vi "AE_Continuous_All.vi"() -> ()   [LabVIEW 2012]
uses:
  <vilib>/DAQmx/read.llb/DAQmx Read (Analog 1D Wfm NChan NSamp).vi
  <vilib>/DAQmx/create/channels.llb/DAQmx Create Channel (AI-Voltage-Basic).vi
  <vilib>/DAQmx/configure/timing.llb/DAQmx Timing (Sample Clock).vi
  <vilib>/DAQmx/miscellaneous.llb/DAQmx Fill In Error Info.vi
panel:
  in  "Physical Channel":tag="Dev1/ai7"
  in  "Gain":u16(ring)=1 items=["20 dB", "40 dB", "60 dB"]
  in  "stop":bool
  in  "Test Name":string="test"
  in  "Storage Directory":path=path "C:/Users/User/Desktop/Users_2013-2014/Michael Rossol"
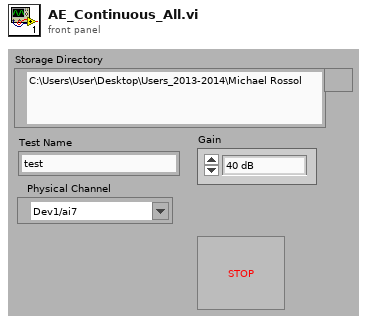
[diagram p1: front panel]
types:
  T1 = enum16{"open", "open or create", "create or replace", "create", "open (read only)"}
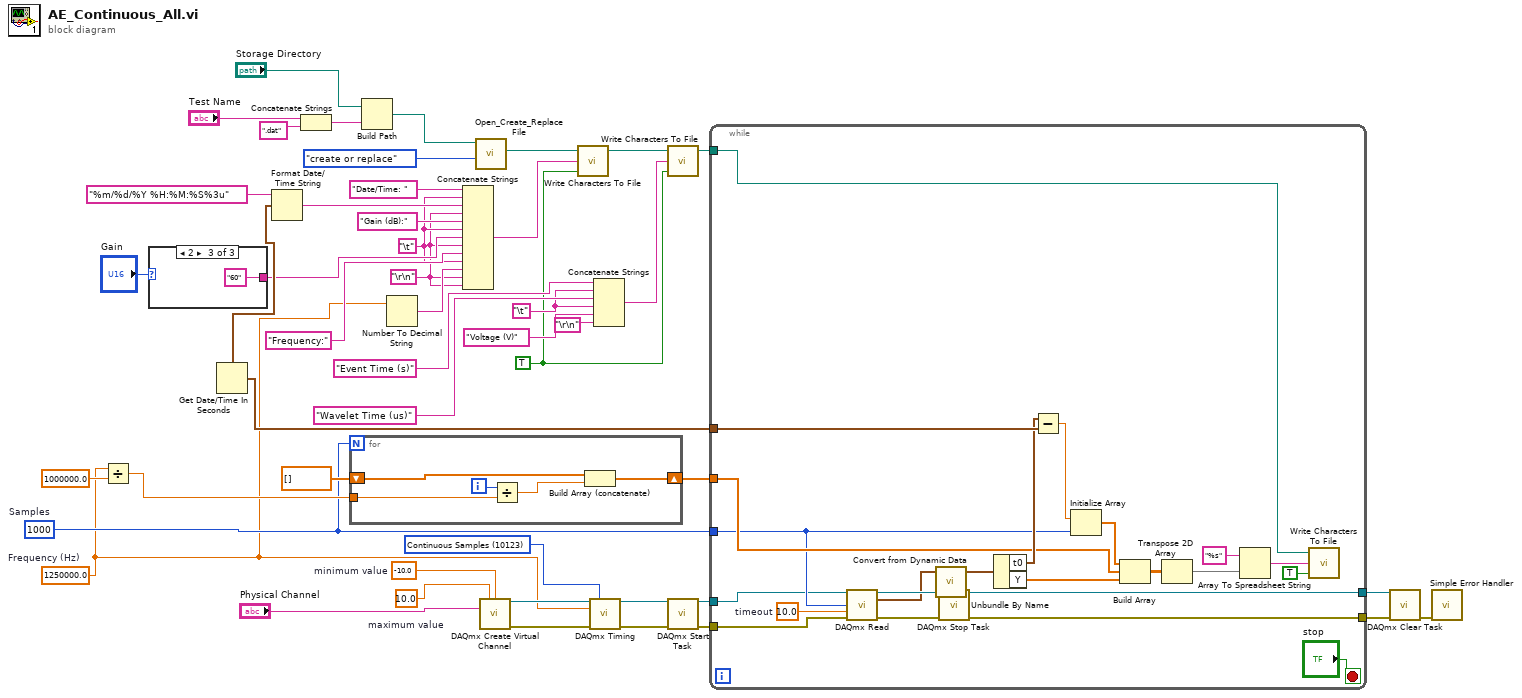
[diagram p0: block diagram]
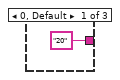
[diagram p2: hidden frame]
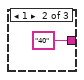
[diagram p3: hidden frame]
diagram:
  w2 = 1000  # Samples
  w20 = -10.0  # minimum value
  w21 = 10.0  # maximum value
  w17 = 10123 items=["Finite Samples"=10178, "Continuous Samples"=10123] ("sample mode")
  w31 = "\t"
  w1 = 1250000.0  # Frequency (Hz)
  w9 = "\t"
  w7 = "\r\n"
  w28 = TRUE ("append to file? (new file:F)")
  n1 = Divide(x=w1, y=1000000.0) -> (x/y=w34:dbl)
  n2 = case shown="2" "Gain" {
    tunnel: ["20" ("string") "40" ("string") "60" ("string")] -> w22
    frame 0, Default {
    }
    frame 1 {
    }
    frame 2 {
    }
  }
  n3 = Get Date/Time In Seconds() -> (seconds since 1Jan1904=w35:timestamp)
  n4 = Format Date/Time String(time format string (%c)="%m/%d/%Y %H:%M:%S%3u", seconds (now)=w35) -> (date/time string=w37:string)  [unwired: 1 in]
  n5 = Concatenate Strings("Test Name", ".dat" ("string")) -> (w40:string)
  n6 = for {
    N: w2 -> [_]
    shift-right: [w54] -> w13
    shift-left: dbl[] [] -> [w55]
    tunnel: w34 -> [w51]
    i -> [w53]
    n7 = Divide(x=w53, y=w51) -> (x/y=w52:dbl)
    n8 = Build Array (concatenate)(w55, w52) -> (w54:dbl[])
  }
  n9 = Build Path(base path="Storage Directory", name or relative path=w40) -> (appended path=w38:path)
  n10 = Number To Decimal String(number=w1) -> (decimal integer string=w8:string)  [unwired: 1 in]
  n11 = Concatenate Strings("Date/Time: ", w9, w37, w7, "Gain (dB):" ("string"), w9, w22, w7, "Frequency:" ("string"), w9, w8, w7, w7) -> (w47:string)
  n12 = call <vilib>:"Open_Create_Replace File.vi"("function (open:0)"=T1."create or replace", "file path"=w38) -> ("new file path"=w43:path)  [unwired: 6 in, 3 out]
  n13 = call-poly <vilib>:"DAQmx Create Virtual Channel.vi"("maximum value"=w21, "minimum value"=w20, "physical channels"="Physical Channel") -> ("task out"=w19:refnum<k21>, "error out"=w18:errorcluster)  [unwired: 11 in]
  n14 = call <vilib>:"Write Characters To File.vi"("append to file? (new file:F)"=w28, "character string"=w47, "file path (dialog if empty)"=w43) -> ("new file path (Not A Path if cancelled)"=w26:path)  [unwired: 2 in]
  n15 = call-poly <vilib>:"DAQmx Timing.vi"("task/channels in"=w19, "sample mode"=w17, "rate"=w1, "error in"=w18) -> ("task out"=w5:refnum<k21>, "error out"=w6:errorcluster)  [unwired: 10 in]
  n16 = Concatenate Strings("Event Time (s)" ("string"), w31, "Wavelet Time (us)" ("string"), w31, "Voltage (V)" ("string"), "\r\n") -> (w27:string)
  n17 = call <vilib>:"Write Characters To File.vi"("append to file? (new file:F)"=w28, "character string"=w27, "file path (dialog if empty)"=w26) -> ("new file path (Not A Path if cancelled)"=w25:path)  [unwired: 2 in]
  n18 = call <vilib>:"DAQmx Start Task.vi"("task/channels in"=w5, "error in"=w6) -> ("task out"=w4:refnum<k21>, "error out"=w3:errorcluster)  [unwired: 12 in]
  n19 = while {
    tunnel: w25 -> [w75]
    tunnel: w2 -> [w59]
    tunnel: w35 -> [w72]
    tunnel: w13 -> [w66]
    tunnel: [w62] -> w15
    tunnel: [w61] -> w14
    tunnel: w4 -> [w57]
    tunnel: w3 -> [w56]
    stop <- "stop" stop-if-true
    w65 = 10.0  # timeout
    n20 = call-poly <vilib>:"DAQmx Read.vi"("task/channels in"=w57, "number of samples per channel"=w59, "timeout"=w65, "error in"=w56) -> ("task out"=w63:refnum<k21>, "data"=w58:waveform(dbl)[], "error out"=w64:errorcluster)  [unwired: 9 in]
    n21 = call "Convert from Dynamic Data"("Dynamic Data Type"=w58) -> ("Waveform"=w73:waveform(dbl))  [unwired: 3 in]
    n22 = call <vilib>:"DAQmx Stop Task.vi"("task/channels in"=w63, "error in"=w64) -> ("task out"=w61:refnum<k21>, "error out"=w62:errorcluster)  [unwired: 12 in]
    n23 = Unbundle By Name(w73) -> ("t0"=w71:timestamp, "Y"=w60:dbl[])
    n24 = Subtract(x=w71, y=w72) -> (x-y=w70:dbl)
    n25 = Initialize Array(w70, w59) -> (w69:dbl[])
    n26 = Build Array(w69, w66, w60) -> (w68:dbl[][])
    n27 = Transpose 2D Array(2D array=w68) -> (transposed array=w67:dbl[][])
    n28 = Array To Spreadsheet String(array=w67, 3:"%s" ("format string")) -> (spreadsheet string=w76:string)  [unwired: 1 in]
    n29 = call <vilib>:"Write Characters To File.vi"("append to file? (new file:F)"=TRUE, "character string"=w76, "file path (dialog if empty)"=w75) -> ()  [unwired: 2 in, 1 out]
  }
  n30 = call <vilib>:"DAQmx Clear Task.vi"("task in"=w14, "error in"=w15) -> ("error out"=w16:errorcluster)  [unwired: 13 in]
  n31 = call <vilib>:"Simple Error Handler.vi"("error in (no error)"=w16) -> ()  [unwired: 4 in, 5 out]
